vi "FinalProject code.vi"() -> ()   [LabVIEW 2016]
uses:
  <vilib>/NXT/NXT Controls/ConnectionType.ctl
  <vilib>/NXT/Block Support/NXT_OutputPort.ctl
  <vilib>/NXT/NXTIO Xnodes/NXTIONodeSubVIs/NXTMotorRunDistance.vi
  <vilib>/NXT/NXTIO Xnodes/AddressXNode/NXTIOAddress.xnode
  <vilib>/NXT/NXTIO Xnodes/NXTIOXNode/NXTIO.xnode
  <vilib>/NXT/Subs/LVHSConnector.ctl
  <vilib>/NXT/LegoClasses/BrickReference/BrickReference.lvclass
panel:
  out "array getting deleted":string[](array[string])
  out "RGB Color":cluster{"Red":u8, "Green":u8, "Blue":u8}
  out "fixed array":string[](array[string])
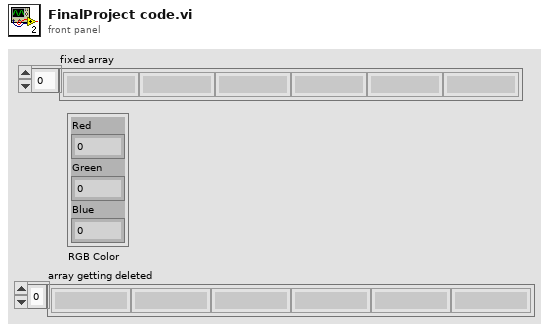
[diagram p1: front panel]
types:
  T1 = typedef "ConnectionType.ctl" = enum16{"Bluetooth", "USB", "WiFi"}
  T2 = typedef "LVHSConnector.ctl" = refnum<class "BrickReference.lvclass">
  T3 = typedef "NXT_OutputPort.ctl" = u8
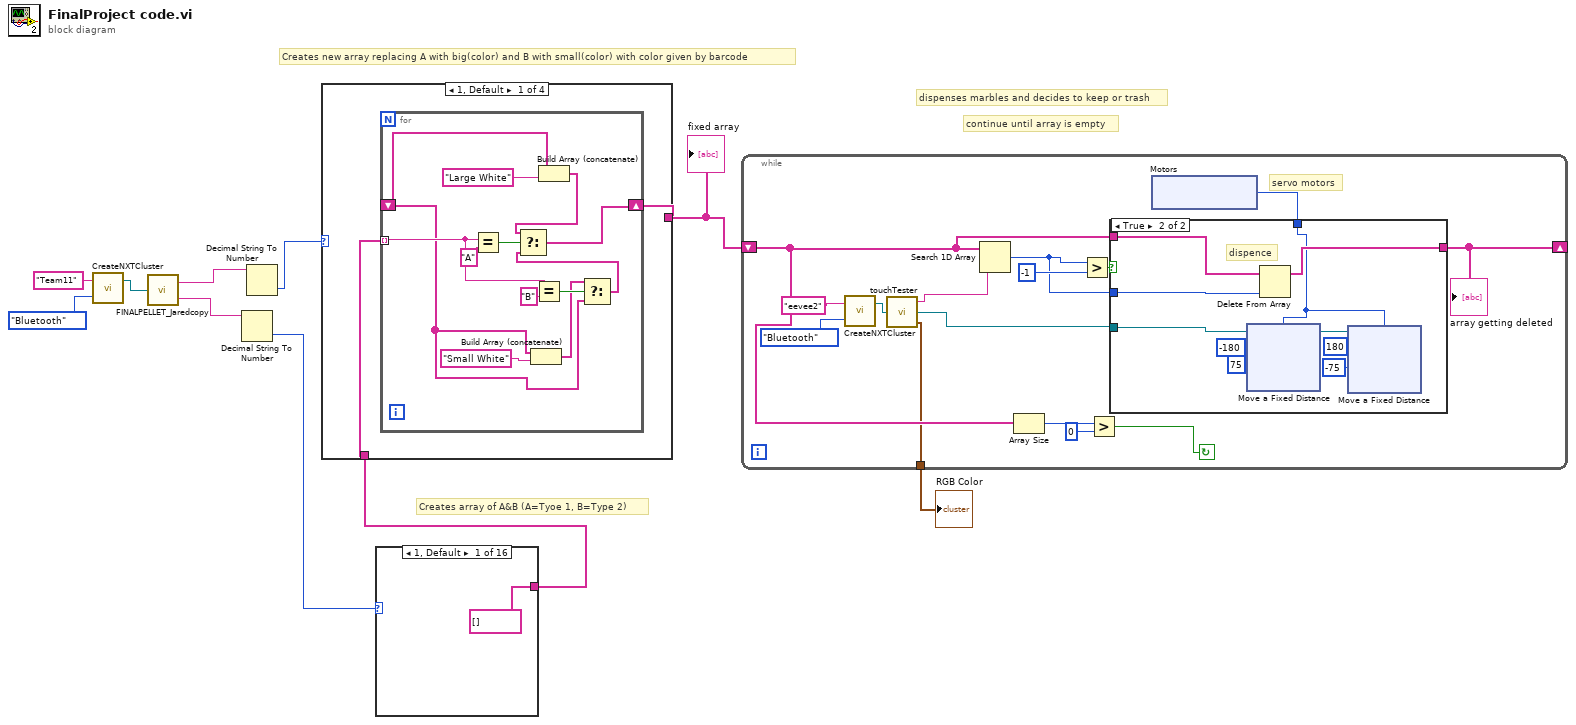
[diagram p0: block diagram]
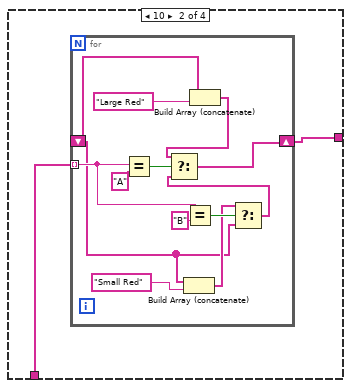
[diagram p2: hidden frame]
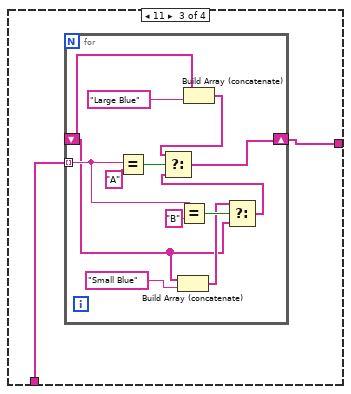
[diagram p3: hidden frame]
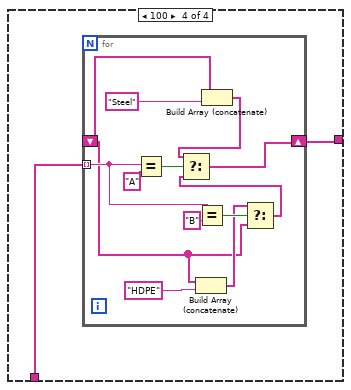
[diagram p4: hidden frame]
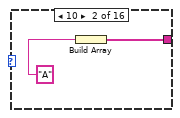
[diagram p5: hidden frame]
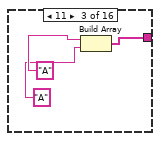
[diagram p6: hidden frame]
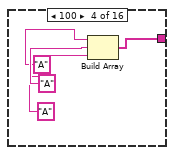
[diagram p7: hidden frame]
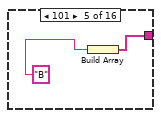
[diagram p8: hidden frame]
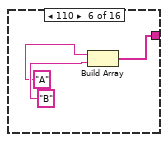
[diagram p9: hidden frame]
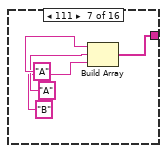
[diagram p10: hidden frame]
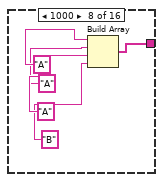
[diagram p11: hidden frame]
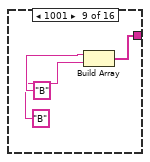
[diagram p12: hidden frame]
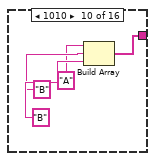
[diagram p13: hidden frame]
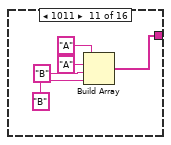
[diagram p14: hidden frame]
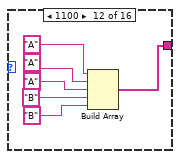
[diagram p15: hidden frame]
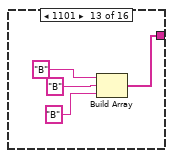
[diagram p16: hidden frame]
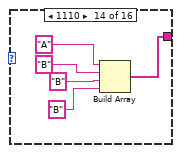
[diagram p17: hidden frame]
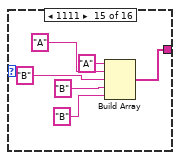
[diagram p18: hidden frame]
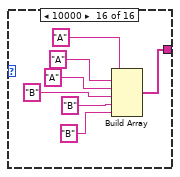
[diagram p19: hidden frame]
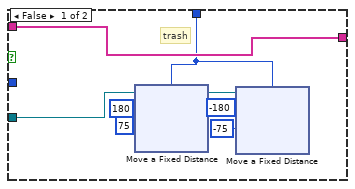
[diagram p20: hidden frame]
diagram:
  # "continue until array is empty"
  # "dispenses marbles and decides to keep or trash"
  # "Creates new array replacing A with big(color) and B with small(color) with color given by barcode"
  # "Creates array of A&B (A=Tyoe 1, B=Type 2)"
  n1 = call <vilib>:"CreateNXTCluster.vi"("Connection Type"=ConnectionType."Bluetooth", "NXT/EV3 name"="Team11") -> ("NXT/EV3"=w6:T2)  [unwired: 2 in]
  n2 = call "FINALPELLET_Jaredcopy.vi"("NXT/EV3"=w6) -> ("Material Binary"=w9:string, "Type Binary"=w10:string)
  n3 = Decimal String To Number(string=w10) -> (number=w2:i32)  [unwired: 2 in, 1 out]
  n4 = Decimal String To Number(string=w9) -> (number=w8:i32)  [unwired: 2 in, 1 out]
  n5 = case shown="1, Default" w2 {
    tunnel: [string[] [] w12 w14 w17 w21 w23 w26 w30 w35 w38 w42 w47 w53 w57 w62 w68] -> w7
    frame 1, Default {
    }
    frame 10 {
      n6 = Build Array("A") -> (w12:string[])
    }
    frame 11 {
      n7 = Build Array("A", "A") -> (w14:string[])
    }
    frame 100 {
      n8 = Build Array("A", "A", "A") -> (w17:string[])
    }
    frame 101 {
      n9 = Build Array("B") -> (w21:string[])
    }
    frame 110 {
      n10 = Build Array("A", "B") -> (w23:string[])
    }
    frame 111 {
      n11 = Build Array("A", "A", "B" ("element")) -> (w26:string[])
    }
    frame 1000 {
      n12 = Build Array("A", "A", "A", "B") -> (w30:string[])
    }
    frame 1001 {
      n13 = Build Array("B", "B") -> (w35:string[])
    }
    frame 1010 {
      n14 = Build Array("A" ("element"), "B", "B") -> (w38:string[])
    }
    frame 1011 {
      n15 = Build Array("A" ("element"), "A" ("element"), "B", "B") -> (w42:string[])
    }
    frame 1100 {
      n16 = Build Array("A" ("element"), "A" ("element"), "A" ("element"), "B", "B") -> (w47:string[])
    }
    frame 1101 {
      n17 = Build Array("B" ("element"), "B", "B") -> (w53:string[])
    }
    frame 1110 {
      n18 = Build Array("A" ("element"), "B" ("element"), "B", "B") -> (w57:string[])
    }
    frame 1111 {
      n19 = Build Array("A" ("element"), "A" ("element"), "B" ("element"), "B", "B") -> (w62:string[])
    }
    frame 10000 {
      n20 = Build Array("A" ("element"), "A" ("element"), "A" ("element"), "B" ("element"), "B", "B") -> (w68:string[])
    }
  }
  n21 = case shown="1, Default" w8 {
    tunnel: w7 -> [w75 w90 w104 w118]
    tunnel: [w76 w89 w103 w117] -> w3
    frame 1, Default {
      n22 = for {
        tunnel: w75 -> [w82] mode=indexing
        shift-right: [w78] -> w76
        shift-left: _ -> [w77]
        n23 = Equal?(x=w82, y="A") -> (x = y?=w88:bool)
        n24 = Build Array (concatenate)(w77, "Small White") -> (w81:string[])
        n25 = Equal?(x=w82, y="B") -> (x = y?=w84:bool)
        n26 = Build Array (concatenate)(w77, "Large White") -> (w85:string[])
        n27 = Select(t=w81, s=w84, f=w77) -> (s? t:f=w79:string[])
        n28 = Select(t=w85, s=w88, f=w79) -> (s? t:f=w78:string[])
      }
    }
    frame 10 {
      n29 = for {
        tunnel: w90 -> [w96] mode=indexing
        shift-right: [w92] -> w89
        shift-left: _ -> [w91]
        n30 = Equal?(x=w96, y="A") -> (x = y?=w102:bool)
        n31 = Build Array (concatenate)(w91, "Small Red") -> (w95:string[])
        n32 = Equal?(x=w96, y="B") -> (x = y?=w98:bool)
        n33 = Build Array (concatenate)(w91, "Large Red") -> (w99:string[])
        n34 = Select(t=w95, s=w98, f=w91) -> (s? t:f=w93:string[])
        n35 = Select(t=w99, s=w102, f=w93) -> (s? t:f=w92:string[])
      }
    }
    frame 11 {
      n36 = for {
        tunnel: w104 -> [w110] mode=indexing
        shift-right: [w106] -> w103
        shift-left: _ -> [w105]
        n37 = Equal?(x=w110, y="A") -> (x = y?=w116:bool)
        n38 = Build Array (concatenate)(w105, "Small Blue") -> (w109:string[])
        n39 = Equal?(x=w110, y="B") -> (x = y?=w112:bool)
        n40 = Build Array (concatenate)(w105, "Large Blue") -> (w113:string[])
        n41 = Select(t=w109, s=w112, f=w105) -> (s? t:f=w107:string[])
        n42 = Select(t=w113, s=w116, f=w107) -> (s? t:f=w106:string[])
      }
    }
    frame 100 {
      n43 = for {
        tunnel: w118 -> [w124] mode=indexing
        shift-right: [w120] -> w117
        shift-left: _ -> [w119]
        n44 = Equal?(x=w124, y="A") -> (x = y?=w130:bool)
        n45 = Build Array (concatenate)(w119, "HDPE") -> (w123:string[])
        n46 = Equal?(x=w124, y="B") -> (x = y?=w126:bool)
        n47 = Build Array (concatenate)(w119, "Steel") -> (w127:string[])
        n48 = Select(t=w123, s=w126, f=w119) -> (s? t:f=w121:string[])
        n49 = Select(t=w127, s=w130, f=w121) -> (s? t:f=w120:string[])
      }
    }
  }
  "fixed array" <- w3
  n50 = while {
    shift-right: [w134] -> _
    shift-left: w3 -> [w135]
    tunnel: [w131] -> w1
    stop <- w138 continue-if-true
    # "servo motors"
    n51 = call <vilib>:"CreateNXTCluster.vi"("Connection Type"=ConnectionType."Bluetooth", "NXT/EV3 name"="eevee2") -> ("NXT/EV3"=w143:T2)  [unwired: 2 in]
    n52 = call "touchTester.vi"("Input"=w143) -> ("String"=w142:string, "NXT/EV3"=w133:T2, "RGB Color"=w131:cluster{"Red":u8, "Green":u8, "Blue":u8})
    n53 = Search 1D Array(1D array=w135, element=w142) -> (index of element=w136:i32)  [unwired: 1 in]
    n54 = Array Size(array=w135) -> (size(s)=w140:i32)
    n55 = Greater?(x=w136, y=-1) -> (0:w137:bool)
    n56 = Greater?(x=w140, y=0) -> (0:w138:bool)
    n57 = xnode "Motors"() -> ("Motor"=w132:T3)
    n58 = case shown="True" w137 {
      tunnel: w136 -> [_ w183]
      tunnel: w135 -> [w154 w184]
      tunnel: [w154 w182] -> w134
      tunnel: w133 -> [w153 w177]
      tunnel: w132 -> [w147 w175]
      frame False {
        # "trash"
        n59 = xnode "Move a Fixed Distance"("Speed 1"=i8 75, "Distance 1"=180, "Motors"=w147, "NXT/EV3"=w153) -> ("NXT/EV3"=w152:T2)
        n60 = xnode "Move a Fixed Distance"("Speed 1"=i8 -75, "Distance 1"=-180, "Motors"=w147, "NXT/EV3"=w152) -> ()  [unwired: 1 out]
      }
      frame True {
        # "dispence"
        n61 = xnode "Move a Fixed Distance"("Speed 1"=i8 75, "Distance 1"=-180, "Motors"=w175, "NXT/EV3"=w177) -> ("NXT/EV3"=w176:T2)
        n62 = Delete From Array(array=w184, index=w183) -> (array with subset deleted=w182:string[])  [unwired: 1 in, 1 out]
        n63 = xnode "Move a Fixed Distance"("Speed 1"=i8 -75, "Distance 1"=180, "Motors"=w175, "NXT/EV3"=w176) -> ()  [unwired: 1 out]
      }
    }
    "array getting deleted" <- w134
  }
  "RGB Color" <- w1
